vi "Set 20 kHz TClk Parameters.vi"(0 "fpga reference in":refnum<k20>[](array[refnum]), 11 "error in":errorcluster) -> (4 "fpga reference out":refnum<k20>[](array[refnum]), 15 "error out":errorcluster)   [LabVIEW 2019]
uses:
  TypeDefs/Shared FPGA Reference.ctl
  <vilib>/Utility/error.llb/Error Cluster From Error Code.vi
  <vilib>/rvi/errors/niLvFpgaAdjustHostInterfaceError.vi
  <vilib>/rvi/interface/nirviReadWriteControl/nirviReadWriteControl.xnode
  <vilib>/rvi/interface/Simulation/niFpgaSimulationCallBeginRW.vi
  NiFpgaLv.dll
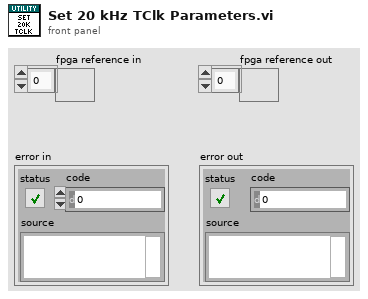
[diagram p1: front panel]
types:
  T1 = typedef "Shared FPGA Reference.ctl" = refnum<k20>
  T2 = typedef "Constants.ctl" = cluster{"data clock rate (Hz)":dbl, "sample rate (Hz)":dbl, "sample rate selector string":string, "default tx bitfile path":path, "default rx bitfile path":path, "default proc bitfile path":path}
  T3 = cluster{"rollover count":u16, "rising edge count":u16, "falling edge count":u16}
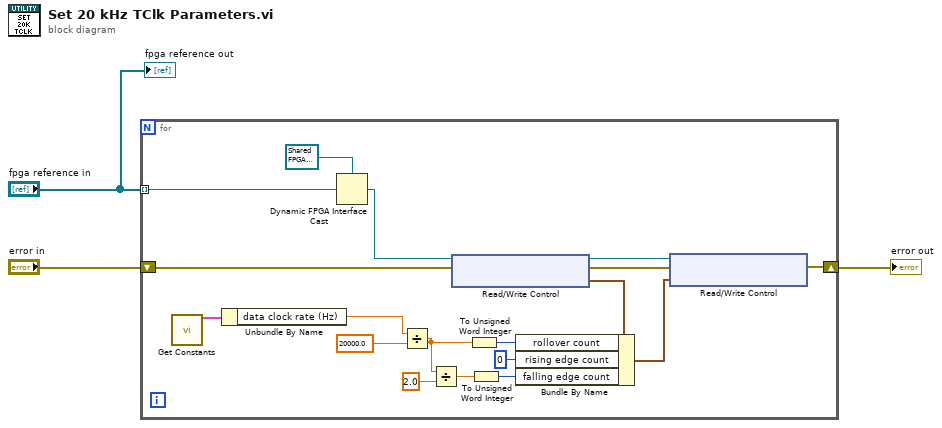
[diagram p0: block diagram]
diagram:
  n1 = for {
    tunnel: "fpga reference in" -> [w18] mode=indexing
    shift-right: [w15] -> w3
    shift-left: "error in" -> [w21]
    n2 = call "Get Constants.vi"() -> ("constants"=w12:T2)  [unwired: 15 in]
    n3 = Unbundle By Name(w12) -> ("data clock rate (Hz)"=w10:dbl)
    n4 = Dynamic FPGA Interface Cast(Session In=T1 refnum ("Refnum in"), Type=w18) -> (Session Out=w20:T1)
    n5 = Divide(x=w10, y=20000.0) -> (x/y=w5:dbl)
    n6 = Divide(x=w5, y=2.0) -> (x/y=w7:dbl)
    n7 = xnode "Read/Write Control"("FPGA VI Reference In"=w20, "error in"=w21) -> ("FPGA VI Reference Out"=w17:T1, "error out"=w16:errorcluster, "20 kHz tclk parameters"=w14:T3)
    n8 = To Unsigned Word Integer(number=w5) -> (unsigned 16bit integer=w8:u16)
    n9 = To Unsigned Word Integer(number=w7) -> (unsigned 16bit integer=w6:u16)
    n10 = Bundle By Name(cluster=w14, "rollover count"=w8, "rising edge count"=u16 0, "falling edge count"=w6) -> (w13:T3)
    n11 = xnode "Read/Write Control"("FPGA VI Reference In"=w17, "error in"=w16, "20 kHz tclk parameters"=w13) -> ("error out"=w15:errorcluster)  [unwired: 1 out]
  }
  "error out" <- w3
  "fpga reference out" <- "fpga reference in"
